vi "流量计UI.vi"() -> ()   [LabVIEW 2016, in "流量计集成.lvlib"]
uses:
  <vilib>/Utility/miscctls.llb/LVPointTypeDef.ctl
  SL1500-3G/UI.vi
  SL1500-3G/SL1500-3G.lvlib
  <vilib>/Utility/config.llb/NI_LVConfig.lvlib
panel:
  in  "返回":bool
  in  "设置":bool
  in  "流量计类型":T1
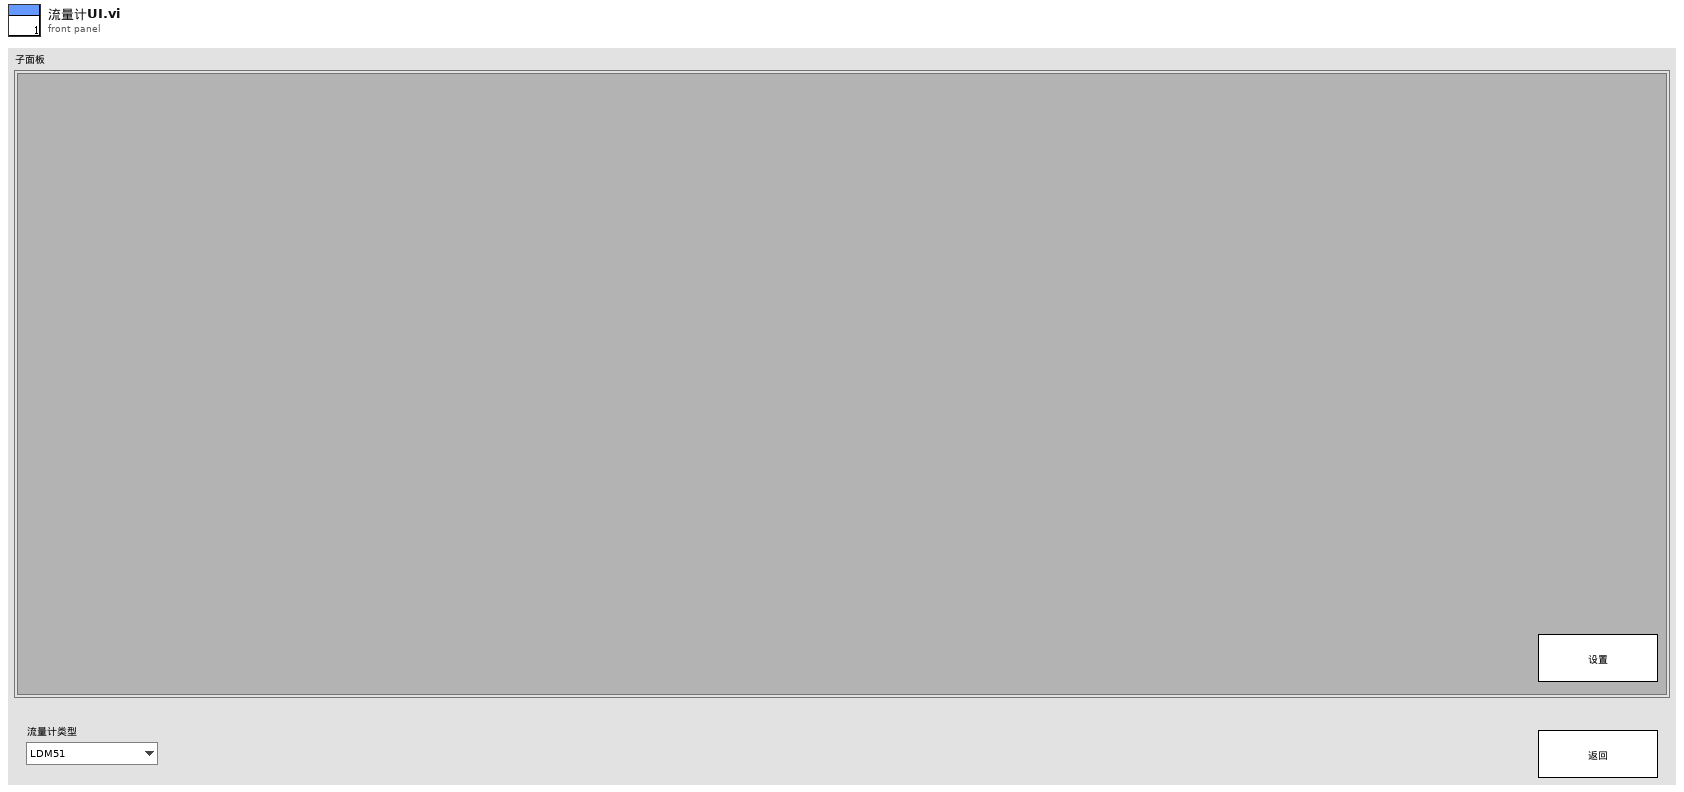
[diagram p1: front panel]
types:
  T1 = typedef "流量计集成.lvlib/流量计类型.ctl" = enum16{"LDM51", "MGG/KL QC", "斯坦道功率测流", "博意达流量计", "SL1500-3G", "WL1A1明渠流量计"}
  T2 = typedef "NI_LVConfig.lvlib/Config Data RefNum.ctl" = refnum<k1>
  T3 = typedef "LVPointTypeDef.ctl" = cluster{"Horizontal":i16, "Vertical":i16}
  T4 = enum32{"Bad", "Idle", "Run top level", "Running"}
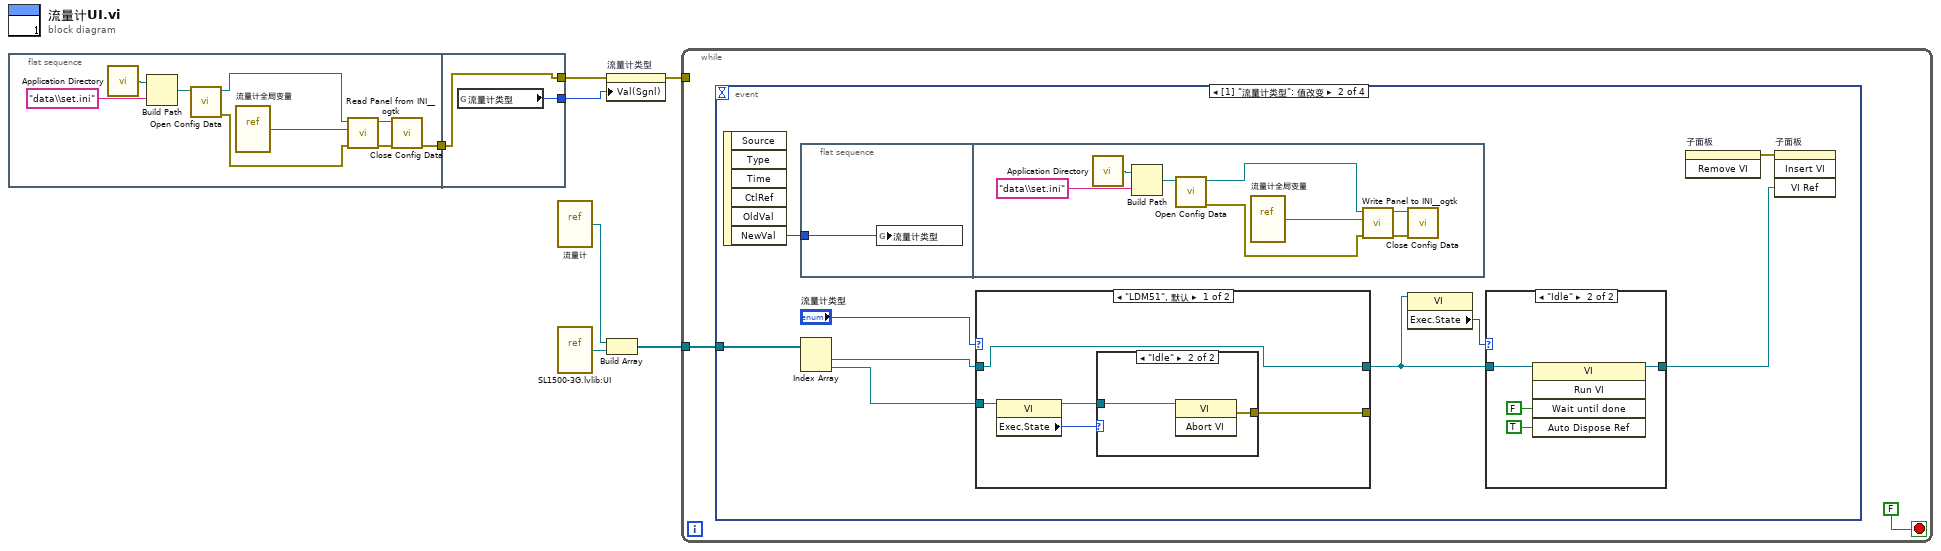
[diagram p0: block diagram]
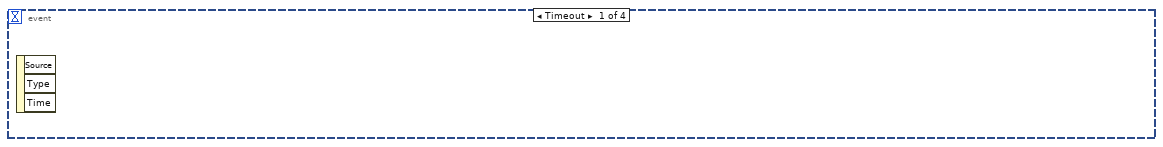
[diagram p2: hidden frame]
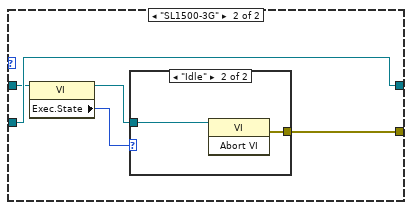
[diagram p5: hidden frame]
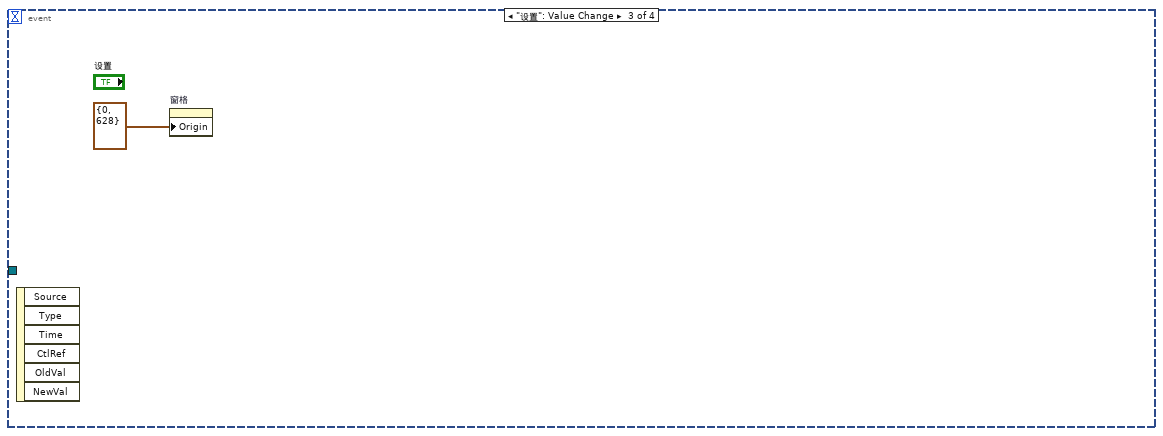
[diagram p7: hidden frame]
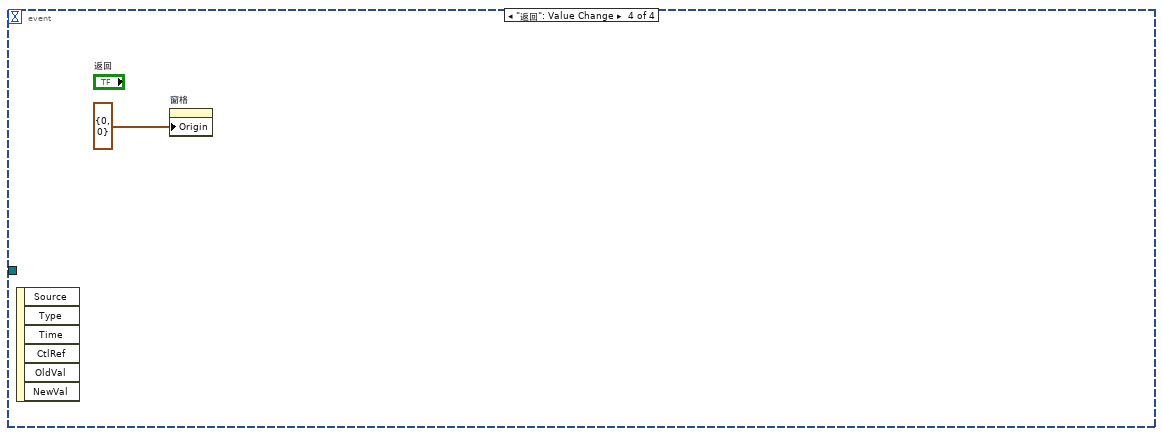
[diagram p8: hidden frame]
diagram:
  n1 = flat-sequence {
    tunnel: [w8] -> w3
    tunnel: w3 -> [w17]
    tunnel: [w18] -> w2
    tunnel: [w17] -> w1
    frame #0 {
      n2 = call <vilib>:"Application Directory.vi"() -> ("Application Directory"=w14:path)
      n3 = Build Path(base path=w14, name or relative path="data\\set.ini" ("名称或相对路径")) -> (appended path=w15:path)
      n4 = call <vilib>:"Open Config Data.vi"("configuration file path"=w15) -> ("error out"=w12:errorcluster, "refnum"=w13:T2)  [unwired: 8 in, 1 out]
      n5 = vi-ref "流量计全局变量.vi"() -> (w9:refnum<vi>)
      n6 = call <userlib>:"Read Panel from INI__ogtk.vi"("error in (no error)"=w12, "VI ref"=w9, "refnum"=w13) -> ("error out"=w10:errorcluster, "refnum out"=w11:T2)  [unwired: 7 in]
      n7 = call <vilib>:"Close Config Data.vi"("error in (no error)"=w10, "refnum"=w11) -> ("error out"=w8:errorcluster)  [unwired: 8 in, 1 out]
    }
    frame #1 {
      n8 = global read "流量计全局变量.vi" "流量计类型"() -> (w18:T1)
    }
  }
  n9 = vi-ref "流量计.vi"() -> (w7:refnum<vi>)
  n10 = vi-ref "SL1500-3G.lvlib:UI.vi"() -> (w6:refnum<vi>)
  n11 = property on="流量计类型" class="Enum (严格)"(error in=w1, "Val(Sgnl)"=w2) -> (error out=w4:errorcluster)  [unwired: 1 in, 1 out]
  n12 = Build Array(w7, w6) -> (w5:refnum<vi>[])
  n13 = while {
    tunnel: w5 -> [w19]
    tunnel: w4 -> [_]
    stop <- FALSE stop-if-true
    n14 = event shown="[1] \"流量计类型\": 值改变" {
      selector: _ -> [_ _ _ _]
      dyn-events: _ -> [_ _ _ _]
      timeout: _ -> [_ _ _ _]
      tunnel: w19 -> [_ w26 _ _]
      event Timeout {
        n15 = event-data() -> ()  [unwired: 1 in, 3 out]
      }
      event Value Change {
        n16 = event-data() -> ("NewVal"=w21:T1)  [unwired: 1 in, 5 out]
        n17 = flat-sequence {
          tunnel: w21 -> [w30]
          frame #0 {
            n18 = global write "流量计全局变量.vi" "流量计类型"(w30) -> ()
          }
          frame #1 {
            n19 = call <vilib>:"Application Directory.vi"() -> ("Application Directory"=w34:path)
            n20 = Build Path(base path=w34, name or relative path="data\\set.ini" ("名称或相对路径")) -> (appended path=w33:path)
            n21 = call <vilib>:"Open Config Data.vi"("configuration file path"=w33) -> ("error out"=w36:errorcluster, "refnum"=w38:T2)  [unwired: 8 in, 1 out]
            n22 = vi-ref "流量计全局变量.vi"() -> (w31:refnum<vi>)
            n23 = call <userlib>:"Write Panel to INI__ogtk.vi"("error in (no error)"=w36, "VI ref"=w31, "refnum"=w38) -> ("error out"=w35:errorcluster, "refnum out"=w37:T2)  [unwired: 7 in]
            n24 = call <vilib>:"Close Config Data.vi"("error in (no error)"=w35, "refnum"=w37) -> ()  [unwired: 8 in, 2 out]
          }
        }
        n25 = Index Array(array=w26) -> (element #1=w25:refnum<vi>, element #2=w24:refnum<vi>)  [unwired: 2 in]
        n26 = case shown="\"LDM51\", 默认" "流量计类型" {
          tunnel: [w48 w55] -> w23
          tunnel: w25 -> [w48 w54]
          tunnel: w24 -> [w47 w55]
          tunnel: [w46 w53] -> _
          frame "LDM51", Default {
            n27 = property class="VI"(reference=w47) -> (reference out=w45:refnum<vi>, "Exec.State"=w44:T4)  [unwired: 1 in, 1 out]
            n28 = case shown="\"Idle\"" w44 {
              tunnel: [_ w50] -> w46
              tunnel: w45 -> [_ w49]
              frame "Bad", Default {
              }
              frame "Idle" {
                n29 = invoke class="VI" method="Abort VI"(reference=w49) -> (error out=w50:errorcluster)  [unwired: 2 in, 2 out]
              }
            }
          }
          frame "SL1500-3G" {
            n30 = property class="VI"(reference=w54) -> (reference out=w52:refnum<vi>, "Exec.State"=w51:T4)  [unwired: 1 in, 1 out]
            n31 = case shown="\"Idle\"" w51 {
              tunnel: [_ w57] -> w53
              tunnel: w52 -> [_ w56]
              frame "Bad", Default {
              }
              frame "Idle" {
                n32 = invoke class="VI" method="Abort VI"(reference=w56) -> (error out=w57:errorcluster)  [unwired: 2 in, 2 out]
              }
            }
          }
        }
        n33 = property class="VI"(reference=w23) -> ("Exec.State"=w22:T4)  [unwired: 1 in, 2 out]
        n34 = case shown="\"Idle\"" w22 {
          tunnel: [w39 w43] -> w28
          tunnel: w23 -> [w39 w40]
          frame "Bad", Default {
          }
          frame "Idle" {
            n35 = invoke class="VI" method="Run VI"(reference=w40, "Wait until done"=FALSE ("结束前等待"), "Auto Dispose Ref"=TRUE ("自动销毁引用")) -> (reference out=w43:refnum<vi>)  [unwired: 2 in, 4 out]
          }
        }
        n36 = invoke on="子面板" class="SubPnl" method="Remove VI"() -> (error out=w29:errorcluster)  [unwired: 3 in, 2 out]
        n37 = invoke on="子面板" class="SubPnl" method="Insert VI"(error in=w29, "VI Ref"=w28) -> ()  [unwired: 2 in, 4 out]
      }
      event "设置": Value Change {
        n38 = event-data() -> ()  [unwired: 1 in, 6 out]
        n39 = property on="窗格" class="Pane"("Origin"=T3 {"Horizontal"=0, "Vertical"=628} ("原点")) -> ()  [unwired: 2 in, 2 out]
      }
      event "返回": Value Change {
        n40 = event-data() -> ()  [unwired: 1 in, 6 out]
        n41 = property on="窗格" class="Pane"("Origin"=T3 {"Horizontal"=0, "Vertical"=0} ("原点")) -> ()  [unwired: 2 in, 2 out]
      }
    }
  }
